vi "tcp_set_mode.vi"(6 "data_in":T1, 8 "error in":errorcluster, 9 "tcp_connected_in":bool, 10 "new_data_available":bool, 11 "connection_id_in":refnum<k5>) -> (0 "error out":errorcluster, 1 "tcp_connected_out":bool, 2 "sva_ready":bool, 3 "connection_id_out":refnum<k5>, 5 "mode_set":bool)   [LabVIEW 2025]
uses:
  28fb5505-a32d-425c-8547-20f3b75436a2.vi
  cda0040a-ea44-4d61-9960-da6bc020597d.vi
  dc8393d8-b758-4f59-8251-f5016f82b5c7.vi
  5675e79b-1a65-4699-bd1f-47e6a3c90739.vi
  70d1167c-81a7-48dc-b05f-7aac217d5c6d.vi
  7bdf989b-3ec4-4ab1-8191-043c43387775.vi
  ffd175c3-585e-4fde-afc2-7d378d641be3.vi
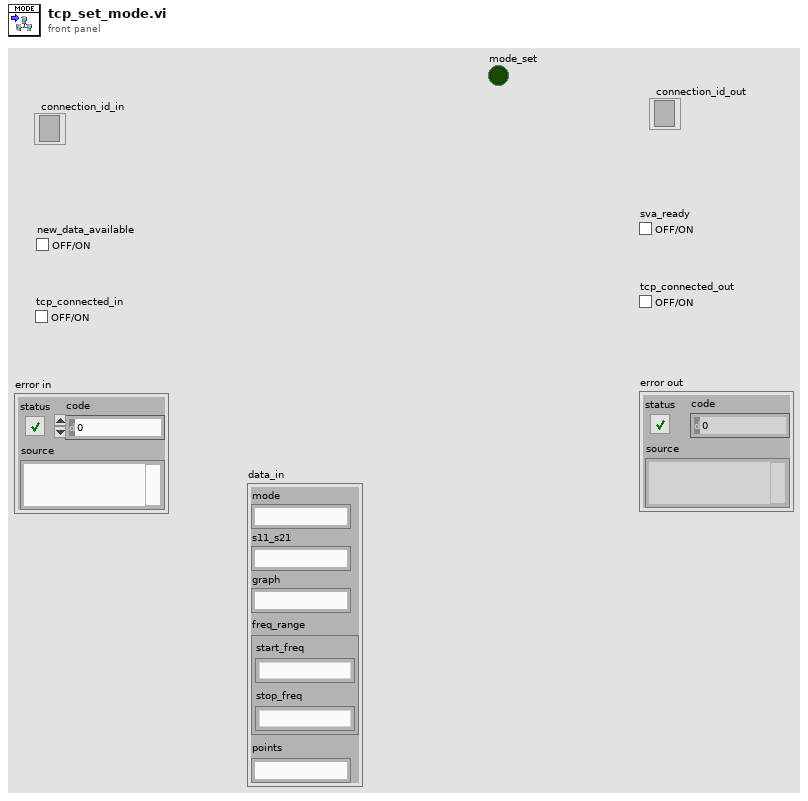
[diagram p1: front panel]
types:
  T1 = cluster{"mode":string, "s11_s21":string, "graph":string, "freq_range":cluster{"start_freq":string, "stop_freq":string}, "points":string}
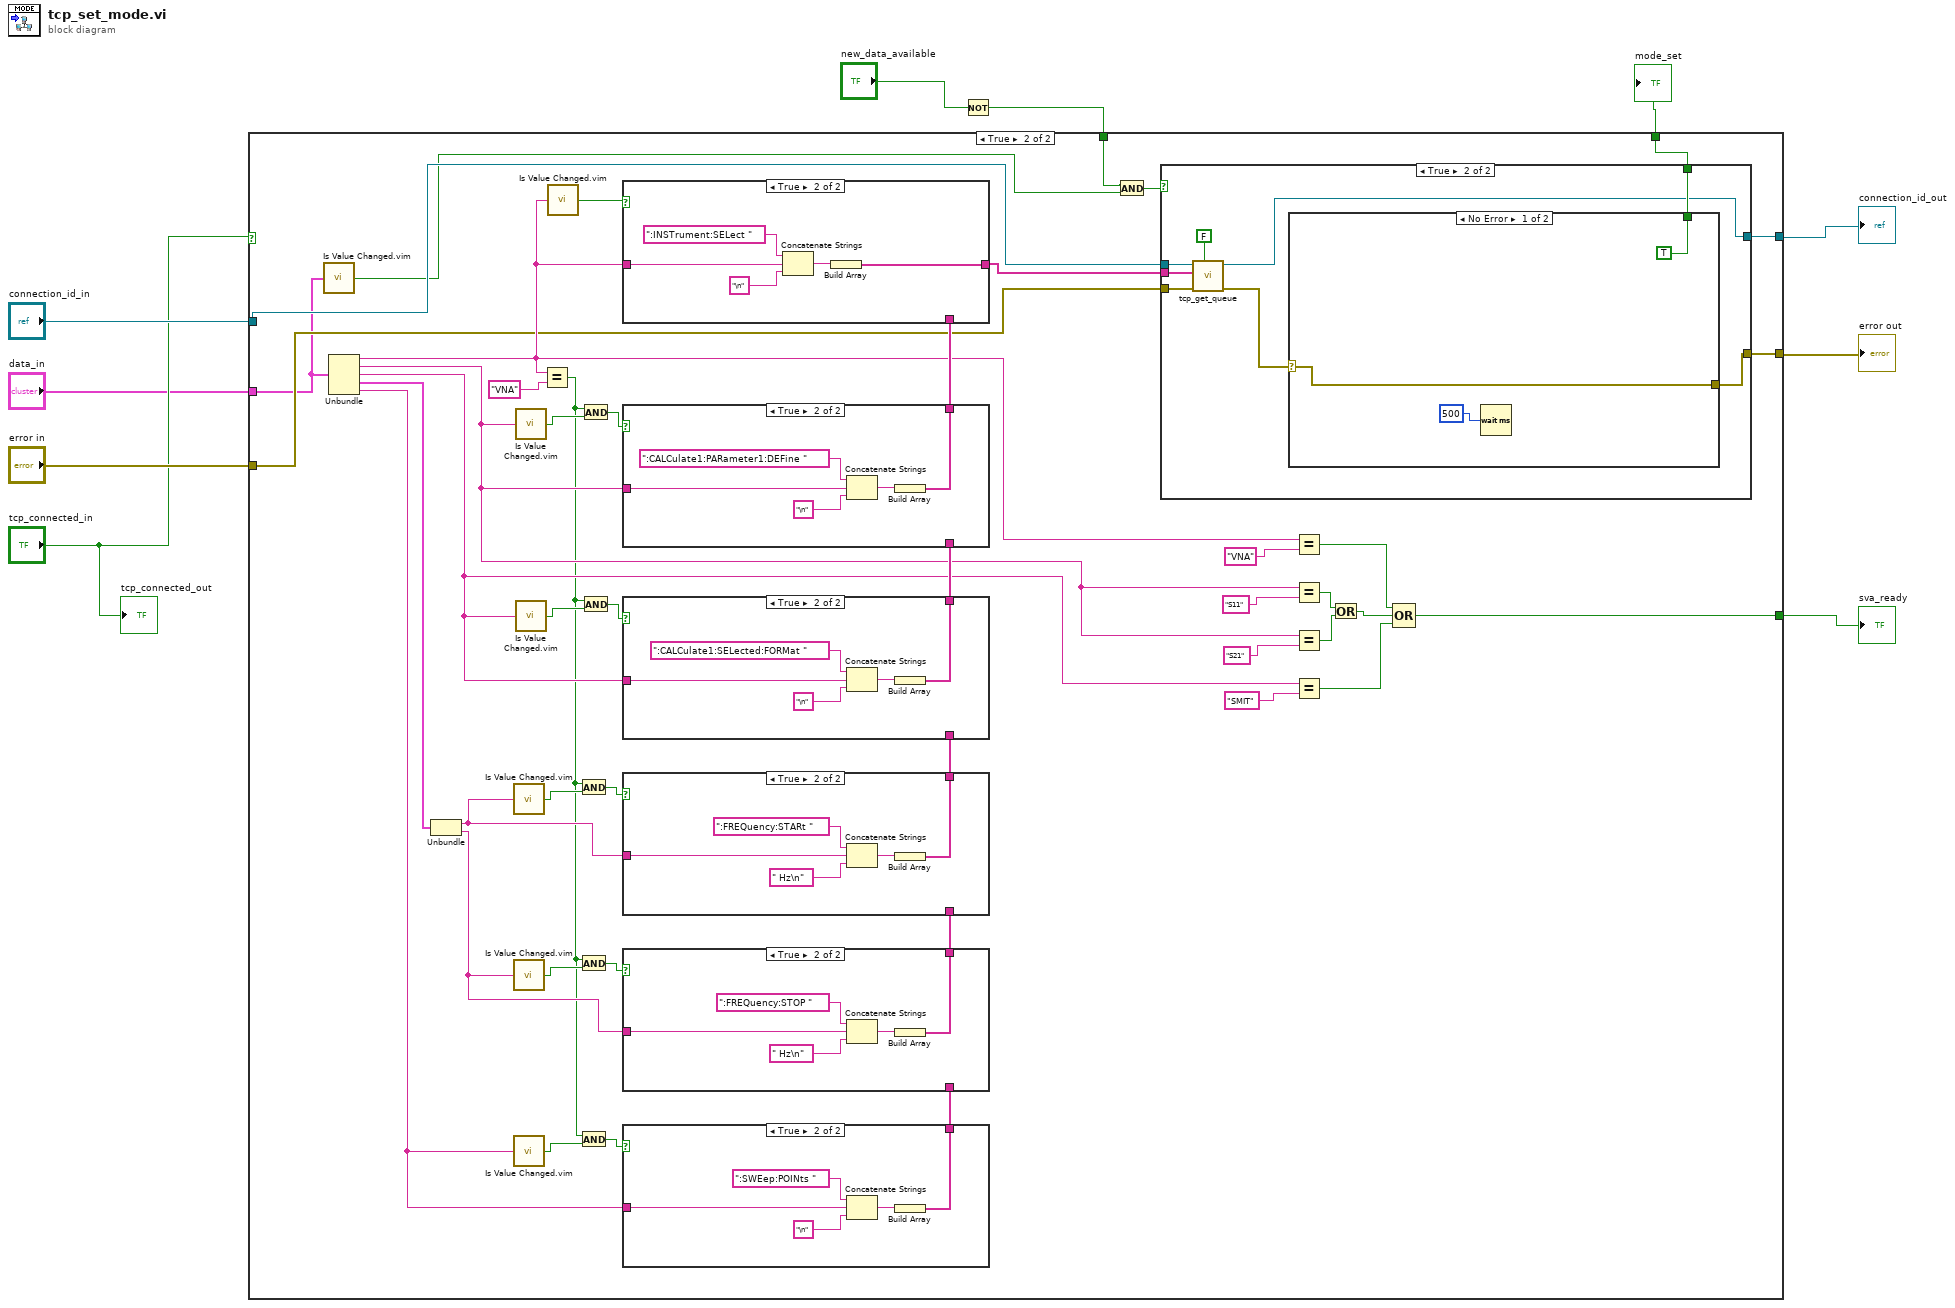
[diagram p0: block diagram]
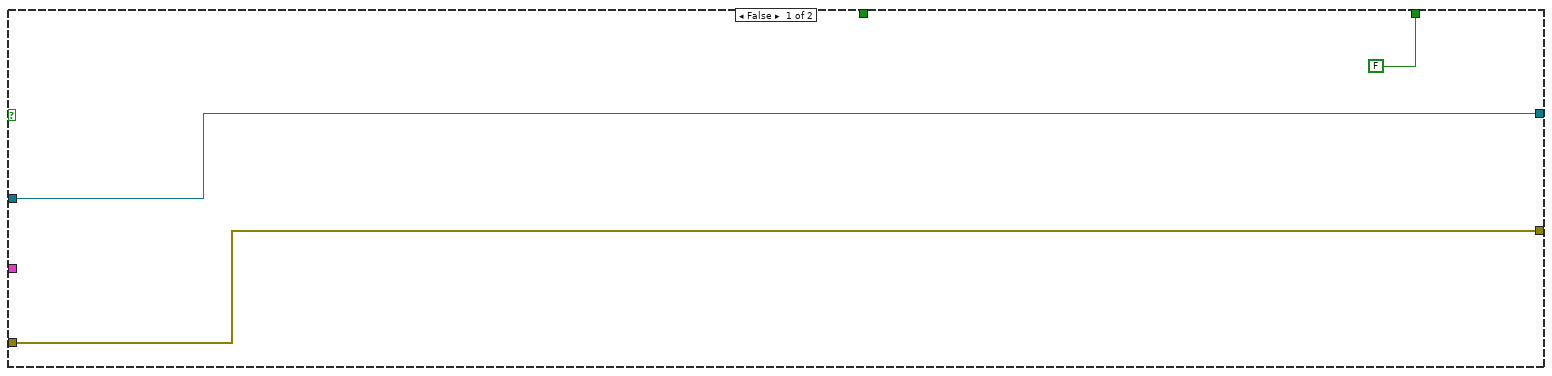
[diagram p2: hidden frame]
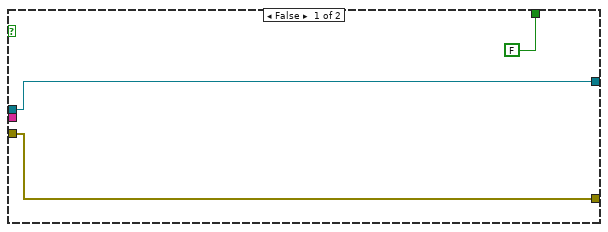
[diagram p6: hidden frame]
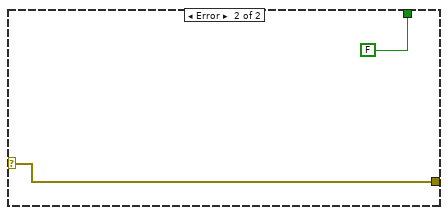
[diagram p7: hidden frame]
diagram:
  n1 = Not(x="new_data_available") -> (.not. x?=w3:bool)
  n2 = case shown="True" "tcp_connected_in" {
    tunnel: [w12 w37] -> w10
    tunnel: [w13 w34] -> w9
    tunnel: "connection_id_in" -> [w13 w51]
    tunnel: "error in" -> [w12 w35]
    tunnel: "data_in" -> [_ w31]
    tunnel: [_ w41] -> w5
    tunnel: [FALSE w36] -> w4
    tunnel: w3 -> [_ w32]
    frame False {
    }
    frame True {
      n3 = call "Is Value Changed.vim"("value"=w31) -> ("changed or first call?"=w30:bool)
      n4 = Unbundle(w31) -> ("mode"=w40:string, "s11_s21"=w39:string, "graph"=w38:string, "freq_range"=w29:cluster{"start_freq":string, "stop_freq":string}, "points"=w16:string)
      n5 = Unbundle(w29) -> ("start_freq"=w24:string, "stop_freq"=w21:string)
      n6 = call "Is Value Changed.vim"("value"=w24) -> ("changed or first call?"=w28:bool)
      n7 = call "Is Value Changed.vim"("value"=w21) -> ("changed or first call?"=w22:bool)
      n8 = call "Is Value Changed.vim"("value"=w16) -> ("changed or first call?"=w18:bool)
      n9 = call "Is Value Changed.vim"("value"=w39) -> ("changed or first call?"=w55:bool)
      n10 = call "Is Value Changed.vim"("value"=w38) -> ("changed or first call?"=w53:bool)
      n11 = Equal?(x=w40, y="VNA") -> (x = y?=w15:bool)
      n12 = call "Is Value Changed.vim"("value"=w40) -> ("changed or first call?"=w58:bool)
      n13 = And(x=w15, y=w28) -> (x .and. y?=w25:bool)
      n14 = And(x=w15, y=w22) -> (x .and. y?=w23:bool)
      n15 = And(x=w15, y=w18) -> (x .and. y?=w17:bool)
      n16 = And(x=w15, y=w55) -> (x .and. y?=w26:bool)
      n17 = And(x=w15, y=w53) -> (x .and. y?=w27:bool)
      n18 = case shown="True" w17 {
        tunnel: [_ w60] -> w14
        tunnel: w16 -> [_ w59]
        frame False {
        }
        frame True {
          n19 = Concatenate Strings(":SWEep:POINts " ("string"), w59, "\n" ("string")) -> (w61:string)
          n20 = Build Array(w61) -> (w60:string[])
        }
      }
      n21 = case shown="True" w23 {
        tunnel: [w64 w66] -> w20
        tunnel: w21 -> [_ w65]
        tunnel: w14 -> [w64 _]
        frame False {
        }
        frame True {
          n22 = Concatenate Strings(":FREQuency:STOP " ("string"), w65, " Hz\n" ("string")) -> (w67:string)
          n23 = Build Array(w67) -> (w66:string[])
        }
      }
      n24 = case shown="True" w25 {
        tunnel: [w70 w72] -> w19
        tunnel: w24 -> [_ w71]
        tunnel: w20 -> [w70 _]
        frame False {
        }
        frame True {
          n25 = Concatenate Strings(":FREQuency:STARt " ("string"), w71, " Hz\n" ("string")) -> (w73:string)
          n26 = Build Array(w73) -> (w72:string[])
        }
      }
      n27 = case shown="True" w27 {
        tunnel: w38 -> [_ w97]
        tunnel: [w92 w93] -> w52
        tunnel: w19 -> [w92 _]
        frame False {
        }
        frame True {
          n28 = Concatenate Strings(":CALCulate1:SELected:FORMat " ("string"), w97, "\n" ("string")) -> (w94:string)
          n29 = Build Array(w94) -> (w93:string[])
        }
      }
      n30 = case shown="True" w26 {
        tunnel: w39 -> [_ w103]
        tunnel: [w98 w99] -> w54
        tunnel: w52 -> [w98 _]
        frame False {
        }
        frame True {
          n31 = Concatenate Strings(":CALCulate1:PARameter1:DEFine " ("string"), w103, "\n" ("string")) -> (w100:string)
          n32 = Build Array(w100) -> (w99:string[])
        }
      }
      n33 = case shown="True" w58 {
        tunnel: w40 -> [_ w109]
        tunnel: [w104 w105] -> w57
        tunnel: w54 -> [w104 _]
        frame False {
        }
        frame True {
          n34 = Concatenate Strings(":INSTrument:SELect " ("string"), w109, "\n" ("string")) -> (w106:string)
          n35 = Build Array(w106) -> (w105:string[])
        }
      }
      n36 = And(x=w32, y=w30) -> (x .and. y?=w33:bool)
      n37 = case shown="True" w33 {
        tunnel: w57 -> [_ w86]
        tunnel: w51 -> [w78 w85]
        tunnel: [w77 w84] -> w37
        tunnel: [FALSE w82] -> w36
        tunnel: w35 -> [w77 w81]
        tunnel: [w78 w80] -> w34
        frame False {
        }
        frame True {
          n38 = call "tcp_get_queue.vi"("response?"=FALSE, "error in"=w81, "command queue"=w86, "connection in"=w85) -> ("error out"=w83:errorcluster, "connection out"=w80:refnum<k5>)  [unwired: 5 in, 1 out]
          n39 = case shown="No Error" w83 {
            selector: w83 -> [w89 w91]
            tunnel: [w89 w91] -> w84
            tunnel: [TRUE FALSE] -> w82
            frame No Error {
              n40 = Wait (ms)(milliseconds to wait=u32 500) -> ()  [unwired: 1 out]
            }
            frame Error {
            }
          }
        }
      }
      n41 = Equal?(x=w40, y="VNA") -> (x = y?=w44:bool)
      n42 = Equal?(x=w39, y="S11") -> (x = y?=w46:bool)
      n43 = Equal?(x=w39, y="S21") -> (x = y?=w45:bool)
      n44 = Equal?(x=w38, y="SMIT") -> (x = y?=w42:bool)
      n45 = Or(x=w46, y=w45) -> (x .or. y?=w43:bool)
      n46 = Compound Arithmetic op=OR(w44, w43, w42) -> (w41:bool)
    }
  }
  "error out" <- w10
  "connection_id_out" <- w9
  "sva_ready" <- w5
  "mode_set" <- w4
  "tcp_connected_out" <- "tcp_connected_in"
